vi "mod_Rayleigh Selective Fading (Jakes).vi"(0 "profile length (samples)":i32=1000, 1 "number of paths":i32=1, 5 "sampling frequency (Hz)":dbl=1.0 format="%.2f", 7 "doppler spread (Hz)":dbl=0.01 format="%.2p", 9 "seed in (0xFFFFFFFF)":i32=-1 format="%.0x", 11 "error in (no error)":errorcluster, 12 "fading variance":dbl=1.0 format="%.2f", 13 "reset? (T)":bool=TRUE) -> (4 "fading profile":cdb[][](array[numeric]), 10 "next seed":i32=-1 format="%.0x", 15 "error out":errorcluster)   [LabVIEW 2020, in "niDMT.lvlib"]
doc: "The Rayleigh fading channel is generated based on Clarke and Gans Model using the Doppler filter with U-shaped power spectral density. \n \n\n Inputs:\n 1) Doppler spread (Hz) \n - range : double precision (default:20)\n - an example : a running vehicle with 65mph (104km/h), the carrier frequency of 900MHz\n The speed of the vehicle = 65*1.6*1000/3600 = 28.89m/s\n Doppler frequency = (900MHz)*(28.89m/s)/(300*10^6m/s) = 86.67 Hz\n 2) Fading variance : the variance of the fading channel output\n - range : double precision (default:2)\n 3) Input waveform : Input signal samples\n - some default values were set.\n (dt:0.00025, the number of samples:4000)\n 4) seed in (0xFFFFFFFF)\n 5) Error in\n\n Outputs:\n 1) Rayleigh fading profile : the complex fading channel output\n 2) Error out"
uses:
  <vilib>/addons/Modulation/niDMT.lvlib
  <vilib>/addons/Modulation/niAMT.lvlib
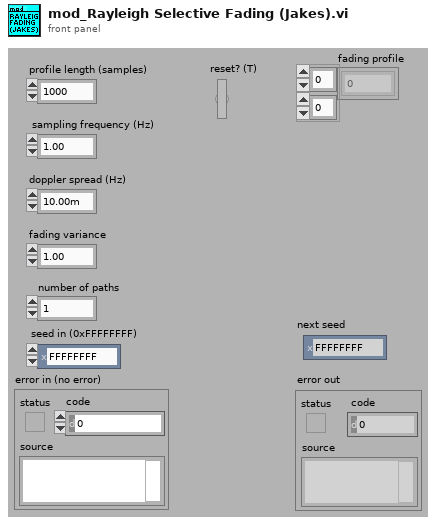
[diagram p1: front panel]
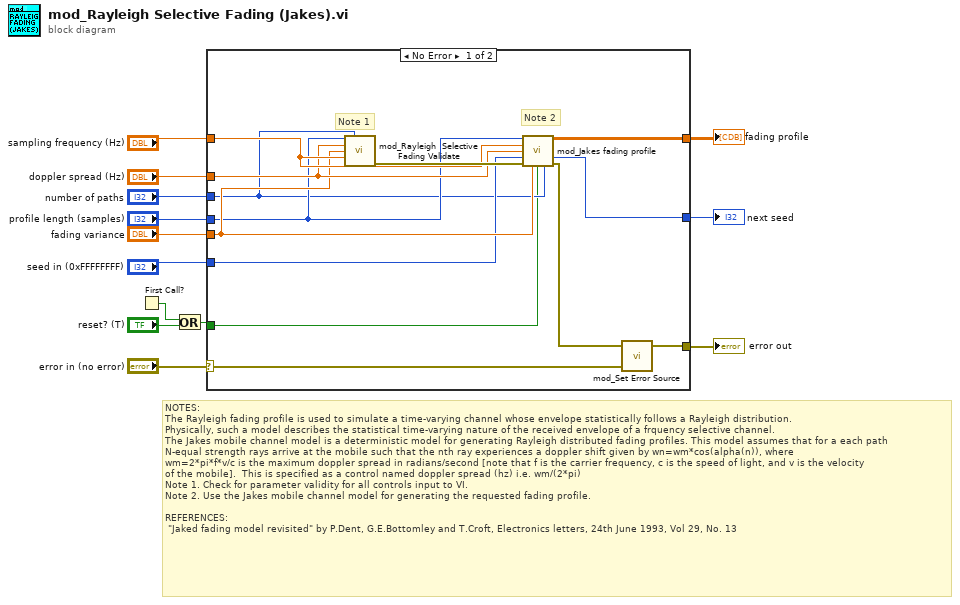
[diagram p0: block diagram]
diagram:
  # "NOTES:\nThe Rayleigh fading profile is used to simulate a time-varying channel whose envelope statistically follows a Rayleigh distribution. \nPhysically, such a model describes the statistical time-varying nature of the received envelope of a frquency selective channel.\nThe Jakes mobile channel model is a deterministic model for generating Rayleigh distributed fading profiles. This model assumes that for a each path\nN-equal strength rays arrive at the mobile such that the nth ray experiences a doppler shift given by wn=wm*cos(alpha(n)), where \nwm=2*pi*f*v/c is the maximum doppler spread in radians/second [note that f is the carrier frequency, c is the speed of light, and v is the velocity \nof the mobile].  This is specified as a control named doppler spread (hz) i.e. wm/(2*pi)\nNote 1. Check for parameter validity for all controls input to VI.\nNote 2. Use the Jakes mobile channel model for generating the requested fading profile.\n\nREFERENCES:\n \"Jaked fading model revisited\" by P.Dent, G.E.Bottomley and T.Croft, Electronics letters, 24th June 1993, Vol 29, No. 13"
  n1 = First Call?() -> (First Call?: T/F=w2:bool)
  n2 = Or(x=w2, y="reset? (T)") -> (x .or. y?=w1:bool)
  n3 = case shown="No Error" "error in (no error)" {
    selector: "error in (no error)" -> [w25 w27]
    tunnel: [w26 w27] -> w13
    tunnel: "sampling frequency (Hz)" -> [w22 _]
    tunnel: "doppler spread (Hz)" -> [w21 _]
    tunnel: "fading variance" -> [w20 _]
    tunnel: "profile length (samples)" -> [w19 _]
    tunnel: "seed in (0xFFFFFFFF)" -> [w18 _]
    tunnel: w1 -> [w14 _]
    tunnel: [w17 _] -> w7
    tunnel: "number of paths" -> [w15 _]
    tunnel: [w16 _] -> w5
    frame No Error {
      # "Note 2"
      # "Note 1"
      n4 = call <vilib>:"mod_Rayleigh  Selective Fading Validate.vi"("profile length (samples)"=w19, "paths"=w15, "doppler spread (Hz)"=w21, "fading variance"=w20, "sampling frequency"=w22) -> ("error out"=w24:errorcluster)  [unwired: 10 out]
      n5 = call <vilib>:"mod_Jakes fading profile.vi"("profile length (samples)"=w19, "sampling frequency (hz)"=w22, "doppler spread (hz)"=w21, "seed in (0xFFFFFFFF)"=w18, "error in (no error)"=w24, "fading variance"=w20, "reset? (T)"=w14, "number of paths"=w15) -> ("fading profile"=w16:cdb[][], "next seed"=w17:i32, "error out"=w23:errorcluster)  [unwired: 5 out]
      n6 = call <vilib>:"mod_Set Error Source.vi"("initial error in (no error)"=w25, "final error in (no error)"=w23) -> ("error out"=w26:errorcluster)  [unwired: 1 in, 2 out]
    }
    frame Error {
    }
  }
  "error out" <- w13
  "next seed" <- w7
  "fading profile" <- w5
